vi "Log Event.vi"(8 "error in (no error)":errorcluster, 10 "String":string, 11 "Controller in":refnum<class "Controller.lvclass">) -> (0 "error out":errorcluster, 3 "Controller out":refnum<class "Controller.lvclass">)   [LabVIEW 2022 SP3, in "Controller.lvlib" / "Controller.lvclass"]
uses:
  Controller.lvclass
  Controller.lvclass/Controller.ctl
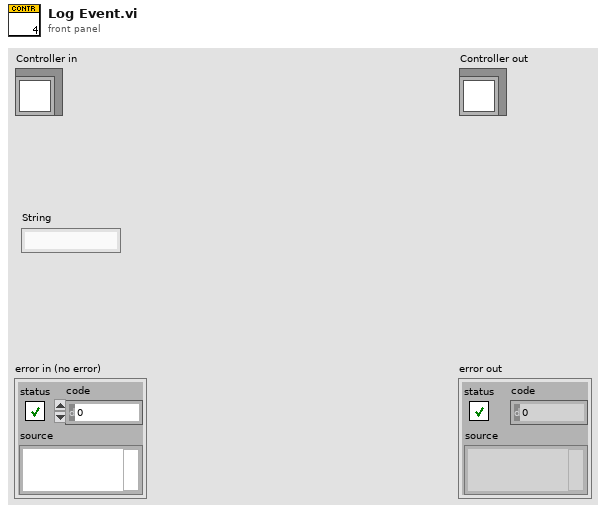
[diagram p1: front panel]
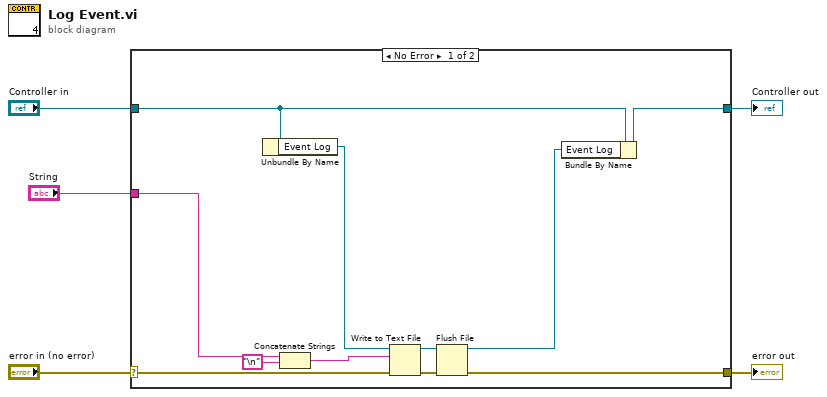
[diagram p0: block diagram]
diagram:
  n1 = case shown="No Error" "error in (no error)" {
    selector: "error in (no error)" -> [w13 w18]
    tunnel: [w10 w18] -> w4
    tunnel: [w14 w17] -> w2
    tunnel: "Controller in" -> [w16 w17]
    tunnel: "String" -> [w11 _]
    frame No Error {
      n2 = Unbundle By Name(w16) -> ("Event Log"=w15:refnum<file>)
      n3 = Concatenate Strings(w11, "\n") -> (w7:string)
      n4 = Write to Text File(file (use dialog)=w15, text=w7, error in=w13) -> (refnum out=w9:refnum<file>, error out=w12:errorcluster)  [unwired: 1 in, 1 out]
      n5 = Flush File(refnum=w9, error in=w12) -> (refnum out=w8:refnum<file>, error out=w10:errorcluster)
      n6 = Bundle By Name(cluster=w16, "Event Log"=w8) -> (w14:refnum<class "Controller.lvclass">)
    }
    frame Error {
    }
  }
  "error out" <- w4
  "Controller out" <- w2
